vi "19-OrientationInfo.vi"(11 "Sensor in":cluster{"Name":string, "Beacons":i32[][]}) -> (3 "Orientation Info":T1)   [LabVIEW 2019, in "19.lvlib"]
uses:
  19.lvlib
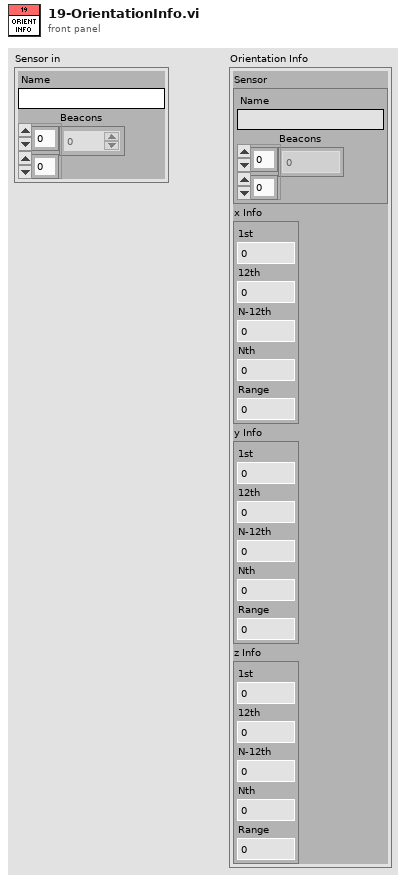
[diagram p1: front panel]
types:
  T1 = cluster{"Sensor":cluster{"Name":string, "Beacons":i32[][]}, "x Info":cluster{"1st":i32, "12th":i32, "N-12th":i32, "Nth":i32, "Range":i32}, "y Info":cluster{"1st":i32, "12th":i32, "N-12th":i32, "Nth":i32, "Range":i32}, "z Info":cluster{"1st":i32, "12th":i32, "N-12th":i32, "Nth":i32, "Range":i32}}
  T2 = cluster{"1st":i32, "12th":i32, "N-12th":i32, "Nth":i32, "Range":i32}
  T3 = cluster{"Sensor in":cluster{"Name":string, "Beacons":i32[][]}, "Axis Info":cluster{"1st":i32, "12th":i32, "N-12th":i32, "Nth":i32, "Range":i32}, "Axis Info":cluster{"1st":i32, "12th":i32, "N-12th":i32, "Nth":i32, "Range":i32}, "Axis Info":cluster{"1st":i32, "12th":i32, "N-12th":i32, "Nth":i32, "Range":i32}}
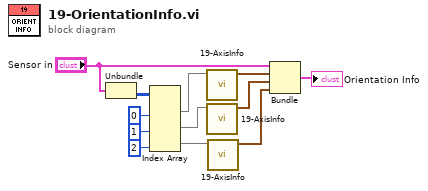
[diagram p0: block diagram]
diagram:
  n1 = Unbundle("Sensor in") -> ("Beacons"=w1:i32[][])  [unwired: 1 out]
  n2 = Index Array(array=w1, index (col) #1=0 ("disabled index (col)"), index (col) #2=1 ("index (col)"), index (col) #3=2 ("index (col)")) -> (element #1=w6:i32[], element #2=w5:i32[], element #3=w4:i32[])  [unwired: 3 in]
  n3 = call "19-AxisInfo.vi"("Axis"=w6) -> ("Axis Info"=w9:T2)  [unwired: 10 in]
  n4 = call "19-AxisInfo.vi"("Axis"=w5) -> ("Axis Info"=w2:T2)  [unwired: 10 in]
  n5 = call "19-AxisInfo.vi"("Axis"=w4) -> ("Axis Info"=w3:T2)  [unwired: 10 in]
  n6 = Bundle("Sensor in"="Sensor in", "Axis Info"=w9, "Axis Info"=w2, "Axis Info"=w3) -> (→"Orientation Info":T3)  [unwired: 1 in]
